vi "TPNT_GetDeviceType.vi"(8 "error in (no error)":errorcluster, 10 "tptype":string, 11 "Object Refnum In":T5) -> (0 "error out":errorcluster, 1 "indexes":i32[](array[numeric]), 2 "Type":T1[](array[typedef]) {"Log"."updaterate" format="%.2f"; "Samples"."Values" format="%.2f"; "Samples"."samples" min=1 step=1; "Limits"."Nominal" format="%.2f"; "Limits"."Upper" format="%.2f"; "Limits"."Lower" format="%.2f"; "update_rate" format="%.2f"}, 3 "Data Refnum out":T5)   [LabVIEW 2016]
uses:
  TPNT_Refnum.ctl
  TPNT_TP.ctl
  TPNT_Limits.ctl
  TPNT_Samples.ctl
  TPNT_Log.ctl
  TPNT_CoreFunction.ctl
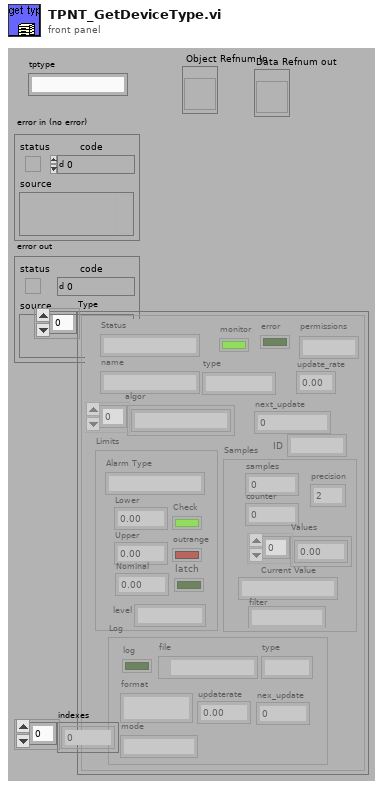
[diagram p1: front panel]
types:
  T1 = typedef "TPNT_TP.ctl" = cluster{"name":string, "type":string, "algor":string[], "update_rate":sgl, "Limits":T2, "Samples":T3, "next_update":u32, "Status":string, "monitor":bool, "error":bool, "Log":T4, "permissions":string, "ID":string}
  T2 = typedef "TPNT_Limits.ctl" = cluster{"Alarm Type":string, "Lower ":dbl, "Upper":dbl, "Nominal":dbl, "outrange":bool, "Check":bool, "latch":bool, "level":string}
  T3 = typedef "TPNT_Samples.ctl" = cluster{"samples":i32, "counter":i32, "Values":dbl[], "Current Value":string, "filter":string, "precision":u8}
  T4 = typedef "TPNT_Log.ctl" = cluster{"log":bool, "file":path, "type":string, "format":string, "updaterate":dbl, "nex_update":u32, "mode":string}
  T5 = typedef "TPNT_Refnum.ctl" = refnum<vi>
  T6 = typedef "TPNT_CoreFunction.ctl" = enum16{"Reset", "Register", "Get Data", "Set Data", "Unregister", "Test", "Get Objects"}
  T7 = typedef "TPNT_DeviceTPs.ctl" = cluster{"device":string, "devupdate":dbl, "next_update":u32, "devinterface":string, "TPs":T1[], "Alarms":bool, "monitor":bool, "log sep":string}
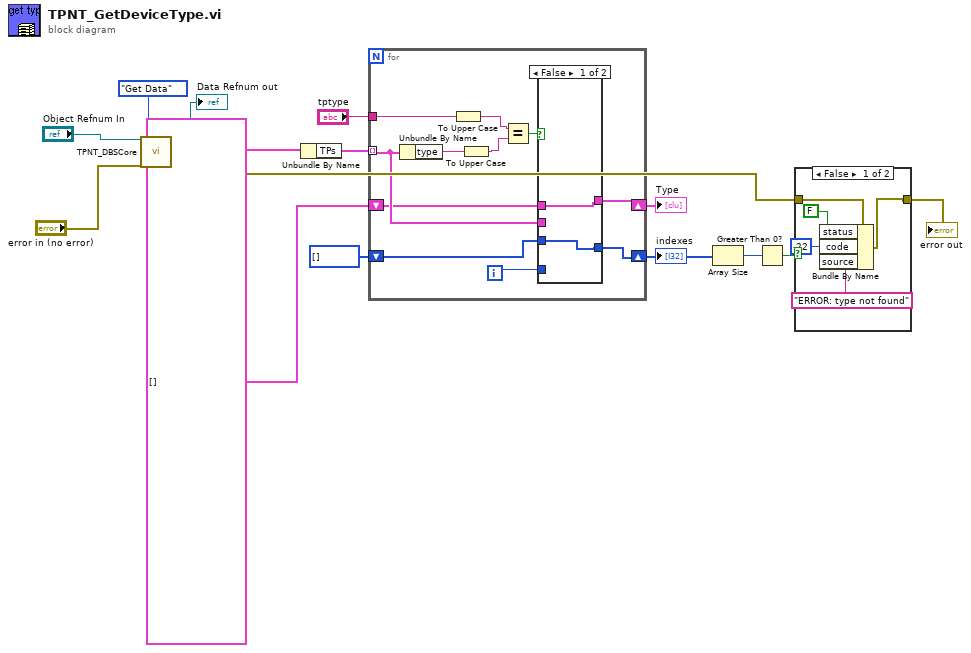
[diagram p0: block diagram]
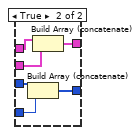
[diagram p3: hidden frame]
diagram:
  n1 = call "TPNT_DBSCore.vi"("Object Refnum In"="Object Refnum In", "error in (no error)"="error in (no error)", "Function (Get Data)"=TPNT_CoreFunction."Get Data") -> ("Object Refnum out"=→"Data Refnum out":T5, "Object Data Out"=w12:T7, "error out"=w4:errorcluster)  [unwired: 2 in, 12 out]
  n2 = Unbundle By Name(w12) -> ("TPs"=w11:T1[])
  n3 = for {
    tunnel: w11 -> [w21] mode=indexing
    tunnel: "tptype" -> [w26]
    shift-right: [w20] -> w7
    shift-left: T1[] [] -> [w19]
    shift-right: [w17] -> w6
    shift-left: i32[] [] -> [w16]
    i -> [w18]
    n4 = Unbundle By Name(w21) -> ("type"=w23:string)
    n5 = To Upper Case(1:w26) -> (0:w25:string)
    n6 = To Upper Case(1:w23) -> (0:w24:string)
    n7 = Equal?(x=w25, y=w24) -> (x = y?=w22:bool)
    n8 = case shown="False" w22 {
      tunnel: w21 -> [_ w34]
      tunnel: [w28 w33] -> w20
      tunnel: w19 -> [w28 w32]
      tunnel: w18 -> [_ w31]
      tunnel: [w27 w30] -> w17
      tunnel: w16 -> [w27 w29]
      frame False {
      }
      frame True {
        n9 = Build Array (concatenate)(w29, w31) -> (w30:i32[])
        n10 = Build Array (concatenate)(w32, w34) -> (w33:T1[])
      }
    }
  }
  "Type" <- w7
  "indexes" <- w6
  n11 = Array Size(array=w6) -> (size(s)=w5:i32)
  n12 = Greater Than 0?(x=w5) -> (x > 0?=w2:bool)
  n13 = case shown="False" w2 {
    tunnel: [w35 w40] -> w3
    tunnel: w4 -> [w39 w40]
    frame False {
      n14 = Bundle By Name(cluster=w39, "status"=FALSE, "code"=-22, "source"="ERROR: type not found") -> (w35:errorcluster)
    }
    frame True {
    }
  }
  "error out" <- w3
